vi "Read System.vi"(8 "error in (no error)":errorcluster, 11 "System configuration in":refnum<class "System configuration.lvclass">) -> (0 "error out":errorcluster, 2 "System":T1={"System Info"={"Project"="", "Program"="W87-1", "Test Name"="No name", "Serial Number"="001", "Plugin"=path "C:/Users/Public/Documents/Sandia National Labs/TSS Plugin", "Glyphs"=path "C:/Users/Public/Documents/Sandia National Labs/Glyphs"}, "Part Info"=0}, 3 "System configuration out":refnum<class "System configuration.lvclass">)   [LabVIEW 2025, in "System.lvlib" / "System configuration.lvclass"]
uses:
  System configuration.lvclass
  System.ctl
  System configuration.lvclass/System configuration.ctl
panel:
  # "Use shorthand name at Test Info"
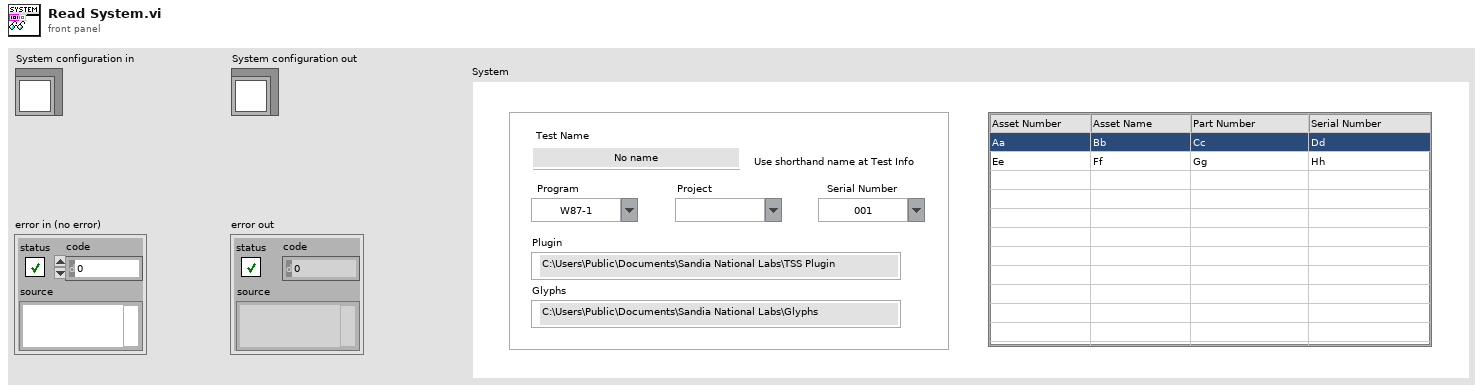
[diagram p1: front panel]
types:
  T1 = typedef "System.lvlib/System configuration.lvclass/System.ctl" = cluster{"System Info":cluster{"Project":string, "Program":string, "Test Name":string, "Serial Number":string, "Plugin":path, "Glyphs":path}, "Part Info":i32}
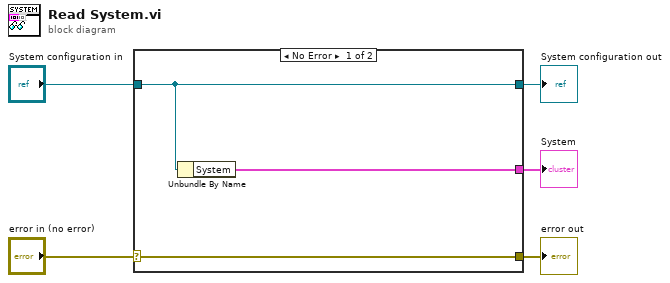
[diagram p0: block diagram]
diagram:
  n1 = case shown="No Error" "error in (no error)" {
    selector: "error in (no error)" -> [w8 w9]
    tunnel: [w8 w9] -> w4
    tunnel: [w7 w10] -> w2
    tunnel: "System configuration in" -> [w7 w10]
    tunnel: [w6 _] -> w1
    frame No Error {
      n2 = Unbundle By Name(w7) -> ("System"=w6:T1)
    }
    frame Error {
    }
  }
  "error out" <- w4
  "System configuration out" <- w2
  "System" <- w1
